vi "Global 9.vi"() -> ()   [LabVIEW 2019]
panel:
  out "Boolean":bool
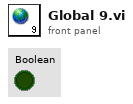
[diagram p1: front panel]
diagram:
